vi "VI Tree.vi"   [LabVIEW 2012, in "Phidget Accelerometer.lvlib"]
doc: "${Accelerometer:VITreeHeader}"
uses:
  <instrlib>/Phidgets/Phidget Accelerometer/Phidget Accelerometer.lvlib
  <instrlib>/Phidgets/Phidget Accelerometer/Public/AccelerometerStart.vi
  <instrlib>/Phidgets/Phidget Accelerometer/Public/AccelerometerOpen.vi
  <instrlib>/Phidgets/Phidget Accelerometer/Public/AccelerometerClose.vi
panel:
  # "(c) 2015 Phidgets Inc..  ALL RIGHTS RESERVED."
  # "SEE DIAGRAM\nFOR VI TREE."
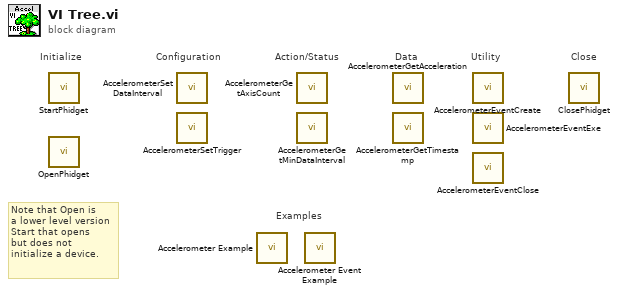
[diagram p0: block diagram]
diagram:
  # "Note that Open is\na lower level version\nStart that opens\nbut does not \ninitialize a device."
  # "Examples"
  # "Configuration"
  # "Utility"
  # "Data"
  # "Action/Status"
  # "Close"
  # "Initialize"
  n1 = call-poly <instrlib>:"StartPhidget.vi"() -> ()  [unwired: 12 in, 4 out]
  n2 = call-poly <instrlib>:"OpenPhidget.vi"() -> ()  [unwired: 8 in, 4 out]
  n3 = call <instrlib>:"AccelerometerSetDataInterval.vi"() -> ()  [unwired: 9 in, 2 out]
  n4 = call <instrlib>:"AccelerometerSetTrigger.vi"() -> ()  [unwired: 9 in, 2 out]
  n5 = call <instrlib>:"Accelerometer Example.vi"() -> ()  [unwired: 12 in]
  n6 = call <instrlib>:"AccelerometerGetAxisCount.vi"() -> ()  [unwired: 8 in, 3 out]
  n7 = call <instrlib>:"AccelerometerGetMinDataInterval.vi"() -> ()  [unwired: 8 in, 3 out]
  n8 = call <instrlib>:"Accelerometer Event Example.vi"() -> ()  [unwired: 12 in]
  n9 = call <instrlib>:"AccelerometerGetAcceleration.vi"() -> ()  [unwired: 8 in, 3 out]
  n10 = call <instrlib>:"AccelerometerGetTimestamp.vi"() -> ()  [unwired: 8 in, 3 out]
  n11 = call <instrlib>:"AccelerometerEventCreate.vi"() -> ()  [unwired: 9 in, 3 out]
  n12 = call <instrlib>:"AccelerometerEventExe.vi"() -> ()  [unwired: 8 in, 8 out]
  n13 = call <instrlib>:"AccelerometerEventClose.vi"() -> ()  [unwired: 10 in, 2 out]
  n14 = call-poly <instrlib>:"ClosePhidget.vi"() -> ()  [unwired: 11 in, 1 out]
